vi "Select Tovey Data.vi"(8 "error in (no error)":errorcluster, 9 "End Time":dbl, 10 "Start Time":dbl, 11 "Model in":refnum<class "Model.lvclass">) -> (0 "error out":errorcluster, 2 "Data":T1[](array[typedef]) {"Timestamp" format="%.4f"; "Mz" format="%.4f"; "My" format="%.4f"; "Mx" format="%.4f"; "Fz" format="%.4f"; "Fy" format="%.4f"; "Fx" format="%.4f"}, 3 "Model out":refnum<class "Model.lvclass">)   [LabVIEW 2016, in "Model.lvclass"]
uses:
  Model.lvclass
  Typedefs/ToveyEngData.ctl
  Model.lvclass/Model.ctl
  Typedefs/FAMT Typedefs.lvlib
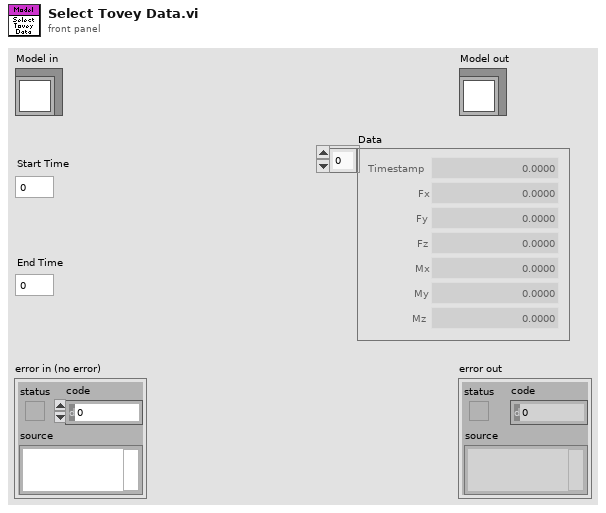
[diagram p1: front panel]
types:
  T1 = typedef "FAMT Typedefs.lvlib/ToveyEngData.ctl" = cluster{"Timestamp":dbl, "Fx":dbl, "Fy":dbl, "Fz":dbl, "Mx":dbl, "My":dbl, "Mz":dbl}
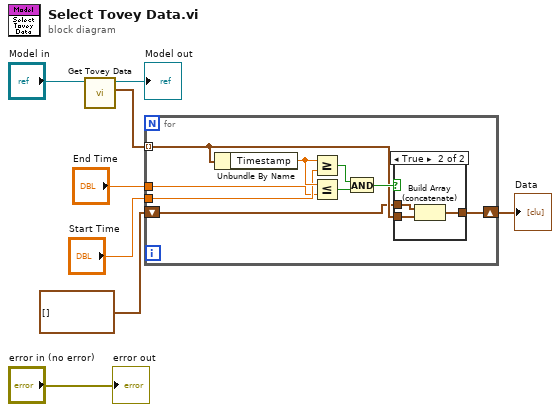
[diagram p0: block diagram]
diagram:
  n1 = call "Get Tovey Data.vi"("Model in"="Model in") -> ("ToveyData"=w7:T1[], "Model out"=→"Model out":refnum<class "Model.lvclass">)  [unwired: 9 in]
  n2 = for {
    tunnel: w7 -> [w13] mode=indexing
    shift-right: [w12] -> w3
    shift-left: T1[] [] -> [w11]
    tunnel: "Start Time" -> [w10]
    tunnel: "End Time" -> [w9]
    n3 = Unbundle By Name(w13) -> ("Timestamp"=w17:dbl)
    n4 = Greater Or Equal?(x=w17, y=w10) -> (x >= y?=w16:bool)
    n5 = Less Or Equal?(x=w17, y=w9) -> (x <= y?=w15:bool)
    n6 = And(x=w16, y=w15) -> (x .and. y?=w14:bool)
    n7 = case shown="True" w14 {
      tunnel: w13 -> [_ w21]
      tunnel: [w18 w20] -> w12
      tunnel: w11 -> [w18 w19]
      frame False {
      }
      frame True {
        n8 = Build Array (concatenate)(w19, w21) -> (w20:T1[])
      }
    }
  }
  "Data" <- w3
  "error out" <- "error in (no error)"
